vi "Send CCD Configuration.vi"(8 "error in (no error)":errorcluster, 11 "Stream in":refnum<class "Stream.lvclass">) -> (0 "error out":errorcluster, 3 "Stream out":refnum<class "Stream.lvclass">)   [LabVIEW 2018, in "Stream.lvclass"]
uses:
  Stream.lvclass
  Stream.lvclass/Stream.ctl
  Interface/Interface.lvclass
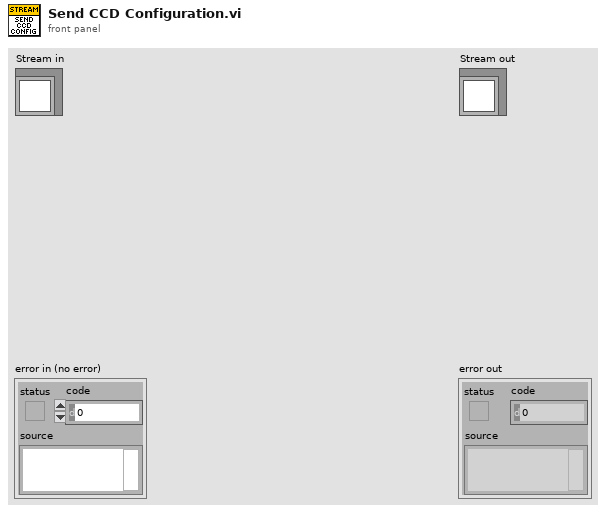
[diagram p1: front panel]
types:
  T1 = cluster{"Exposure Time":sgl, "Pre-amp gain":u8, "Readout Rate":u8, "EM Mode":u8, "EM Gain":u16, "Binning":u16, "Initial Line":u16, "Initial Cloumn":u16, "Final Line":u16, "Final Column":u16, "Kinetic Series Length":u32, "Shutter Mode":u8, "Cooler ON/OFF":u16, "Temperature":i8, "Image Name":string, "Image Path":string, "#Images":u32}
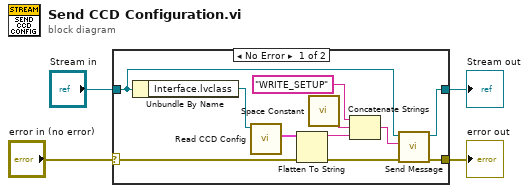
[diagram p0: block diagram]
diagram:
  n1 = case shown="No Error" "error in (no error)" {
    selector: "error in (no error)" -> [w10 w17]
    tunnel: [w6 w17] -> w3
    tunnel: [w9 w16] -> w1
    tunnel: "Stream in" -> [w8 w16]
    frame No Error {
      n2 = Unbundle By Name(w8) -> ("Interface.lvclass"=w15:refnum<class "Interface.lvclass">)
      n3 = call "Read CCD Config.vi"("Interface in"=w15) -> ("CCD Config"=w14:T1)  [unwired: 8 in, 2 out]
      n4 = Flatten To String(anything=w14, error in (no error)=w10) -> (data string=w11:string, error out=w7:errorcluster)  [unwired: 2 in, 1 out]
      n5 = call <vilib>:"Space Constant.vi"() -> ("String"=w12:string)
      n6 = Concatenate Strings("WRITE_SETUP", w12, w11) -> (w5:string)
      n7 = call "Send Message.vi"("error in (no error)"=w7, "Message"=w5, "Stream in"=w8) -> ("error out"=w6:errorcluster, "Stream out"=w9:refnum<class "Stream.lvclass">)  [unwired: 7 in]
    }
    frame Error {
    }
  }
  "error out" <- w3
  "Stream out" <- w1
